vi "endCommunication.vi"(0 "Show Terminal":bool, 1 "Encoder COM Port":refnum<visa-resource-name>) -> ()   [LabVIEW 2020]
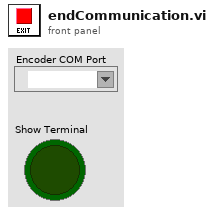
[diagram p1: front panel]
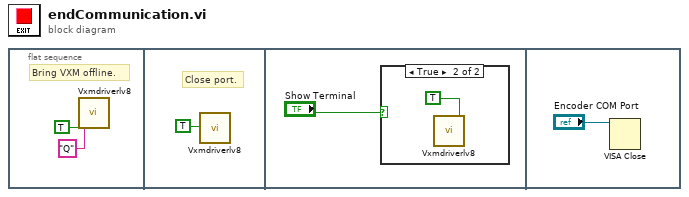
[diagram p0: block diagram]
diagram:
  n1 = flat-sequence {
    frame #0 {
      # "Bring VXM offline."
      n2 = call "Vxmdriverlv8.Vi"("Send\nchars\nto port"=TRUE ("Send\nchars\nto port"), "Chars to send"="Q") -> ()  [unwired: 20 in, 6 out]
    }
    frame #1 {
      # "Close port."
      n3 = call "Vxmdriverlv8.Vi"("Close Port"=TRUE) -> ()  [unwired: 21 in, 6 out]
    }
    frame #2 {
      n4 = case shown="True" "Show Terminal" {
        frame False {
        }
        frame True {
          n5 = call "Vxmdriverlv8.Vi"("Hide Terminal"=TRUE) -> ()  [unwired: 21 in, 6 out]
        }
      }
    }
    frame #3 {
      n6 = VISA Close(VISA resource name="Encoder COM Port") -> ()  [unwired: 1 in, 1 out]
    }
  }
